vi "uDaq.vi"() -> (0 "error out":errorcluster)   [LabVIEW 2017]
uses:
  <vilib>/Platform/TimedLoop/XDataNode/timing_clust.ctl
  <vilib>/Platform/TimedLoop/XDataNode/nitl_modes.ctl
  <vilib>/Platform/TimedLoop/XDataNode/wakeup.ctl
  Globals/measurementGlobal.vi
  <vilib>/platform/TimedLoop/XDataNode/XDataNode.xnode
  <vilib>/Platform/TimedLoop/XDataNode/XDNodeRunTimeDep.lvlib
panel:
  out "Analogue Data (volts?)":dbl[][](array[numeric])
  out "Block Index":i32
  out "Case":string[](array[string])
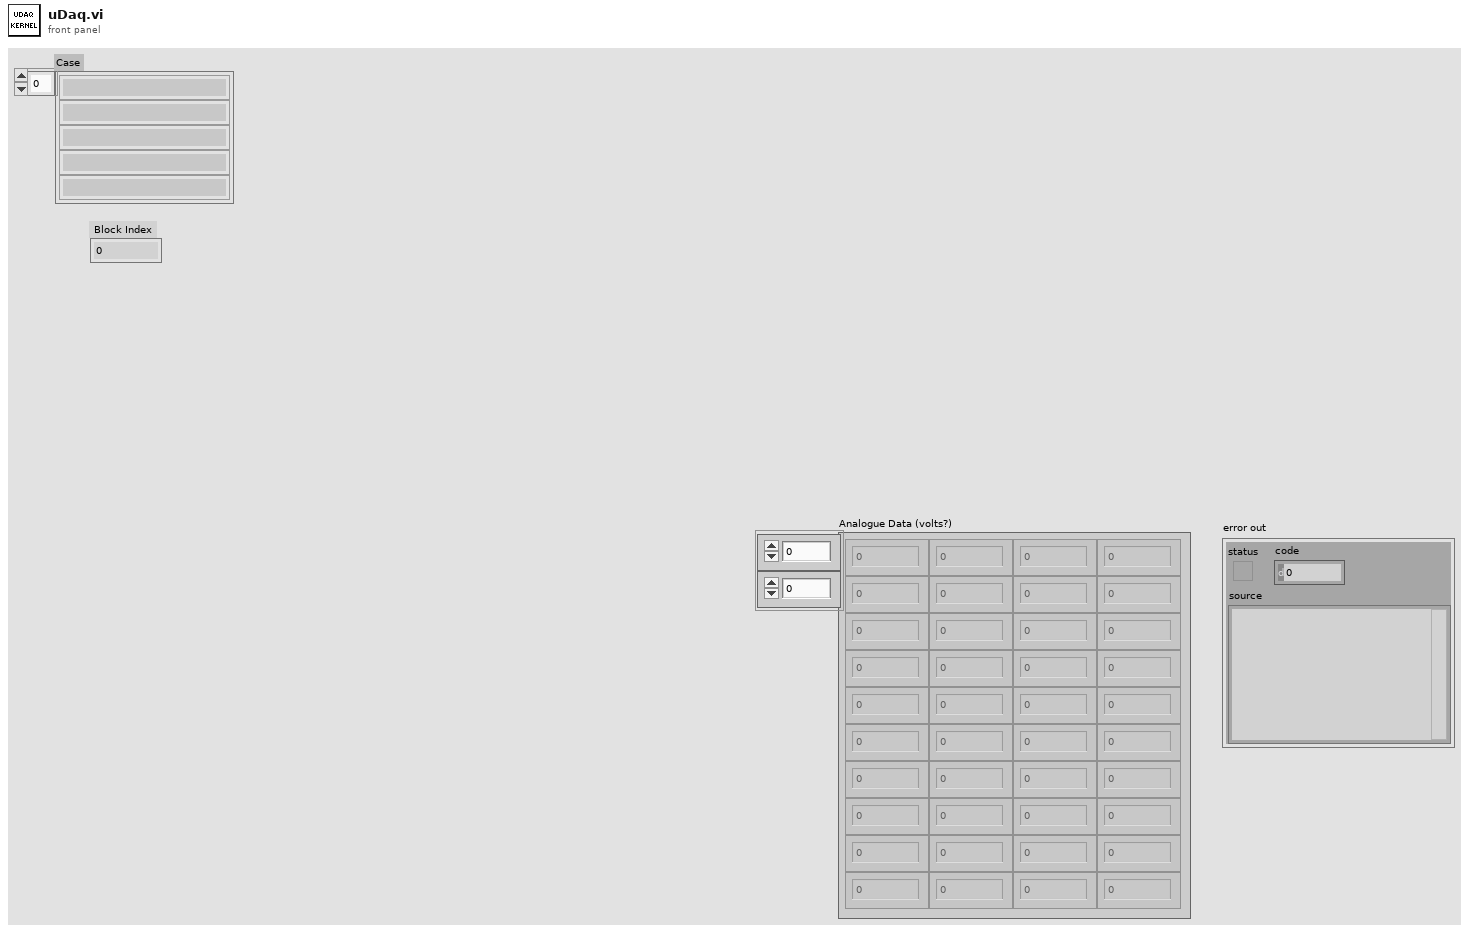
[diagram p1: front panel]
types:
  T1 = typedef "XDNodeRunTimeDep.lvlib/timing_clust.ctl" = cluster{"Expected End [f-1]":u64, "Actual End [f-1]":u64, "Finished Late? [f-1]":bool, "Expected End [i-1]":u64, "Actual End [i-1]":u64, "Finished Late? [i-1]":bool, "Expected Start [i]":u64, "Actual Start [i]":u64, "Expected Start [f]":u64, "Actual Start [f]":u64, "Source Name":string, "Structure Name":string, "Period":i64, "Deadline":i64, "Offset":i64, "Start":i64, "Priority":i32, "Timeout":i32, "Mode":T2, "Wakeup Reason":T3, "Error":errorcluster, "Source Type":string, "Secondary Source Type":string, "Global End Time":u64, "Global Start Time":u64, "Frame Duration":u64, "Iteration Duration":u64, "Assigned CPU":i32, "I/O Scan Engine Mode":u32}
  T2 = typedef "XDNodeRunTimeDep.lvlib/nitl_modes.ctl" = enum32{"No Change", "Process missed periods, maintain original phase", "Discard missed periods, maintain original phase", "Process missed periods, ignore original phase", "Discard missed periods, ignore original phase"}
  T3 = typedef "XDNodeRunTimeDep.lvlib/wakeup.ctl" = enum32{"Normal", "Aborted", "Asynchronous wakeup", "Timing source error", "Timed loop error", "Timeout"}
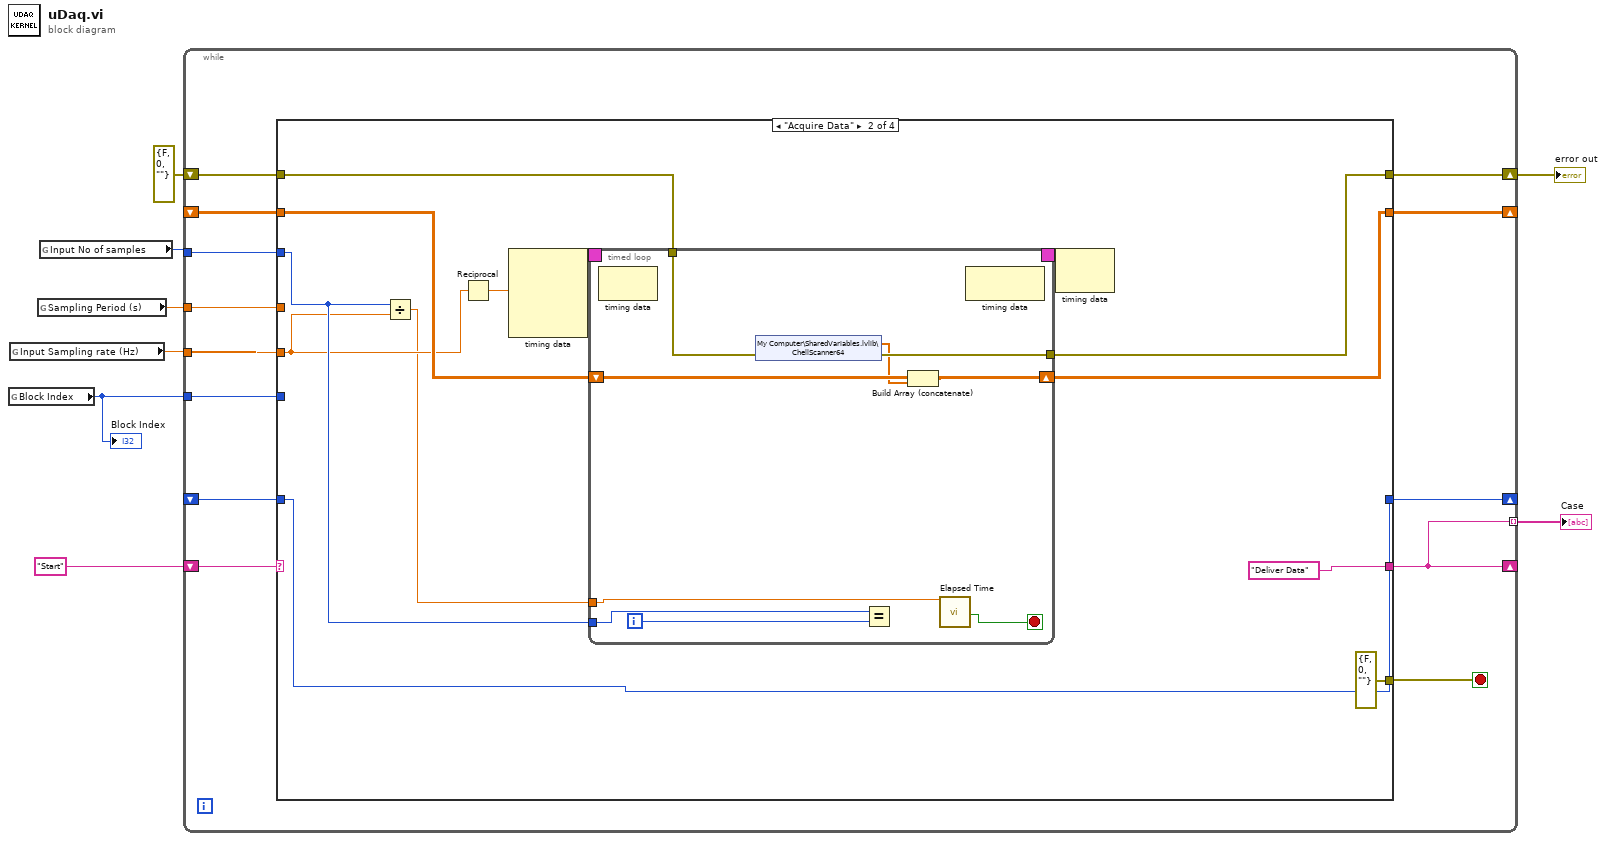
[diagram p0: block diagram]
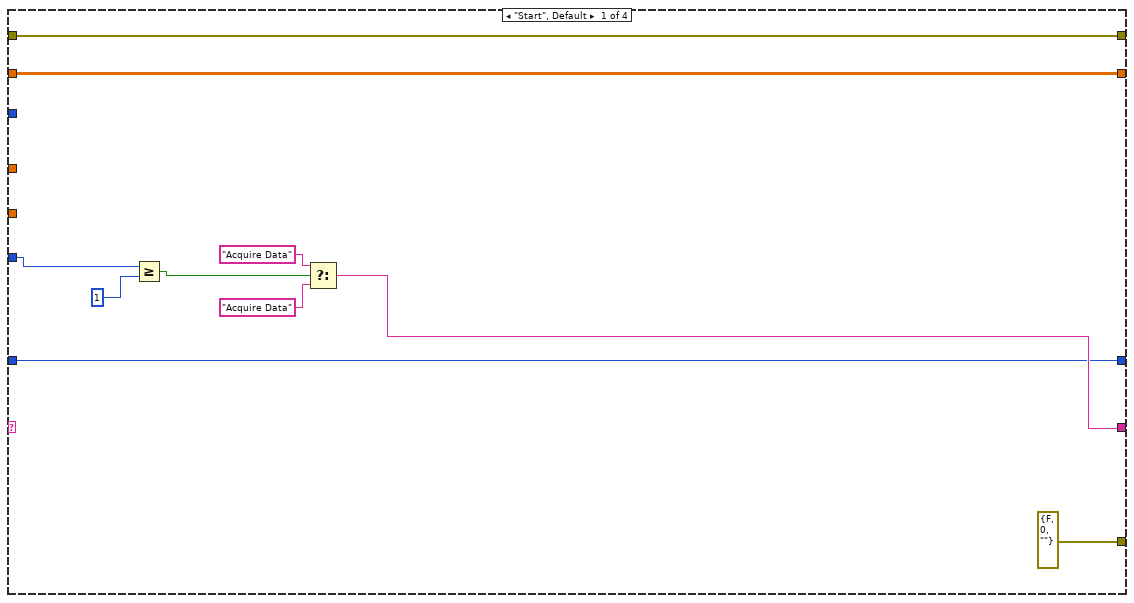
[diagram p2: hidden frame]
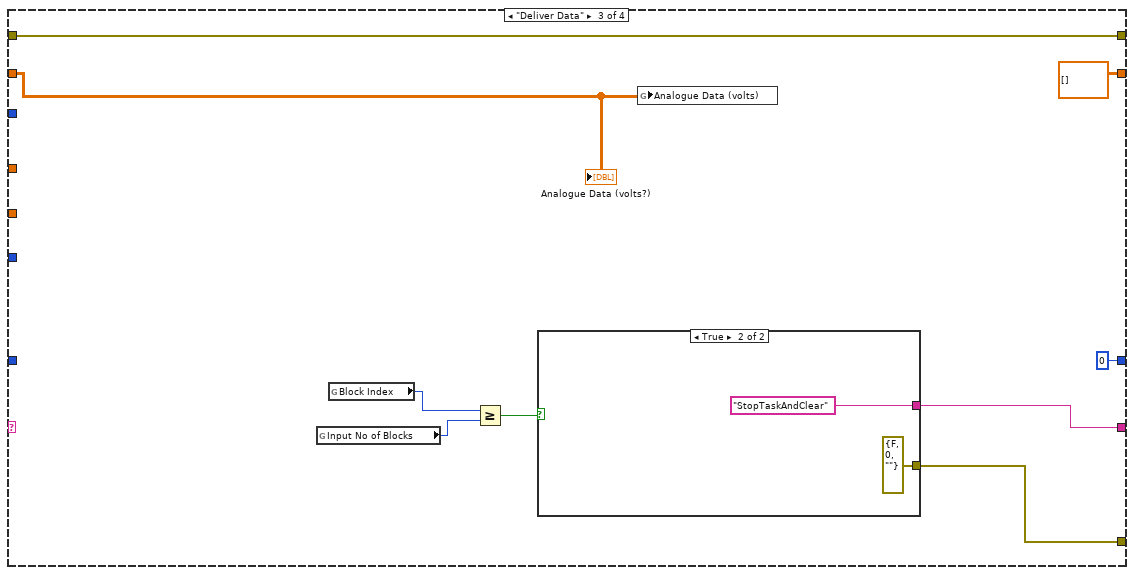
[diagram p3: hidden frame]
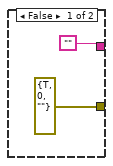
[diagram p4: hidden frame]
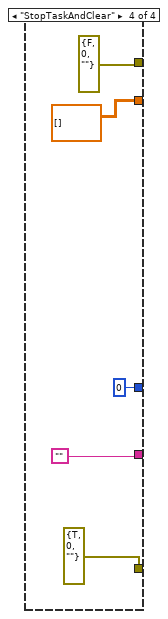
[diagram p5: hidden frame]
diagram:
  n1 = global read "measurementGlobal.vi" "Block Index"() -> (w2:i32)
  "Block Index" <- w2
  n2 = global read "measurementGlobal.vi" "Input Sampling rate (Hz)"() -> (w7:dbl)
  n3 = global read "measurementGlobal.vi" "Sampling Period (s)"() -> (w3:dbl)
  n4 = global read "measurementGlobal.vi" "Input No of samples"() -> (w8:i32)
  n5 = while {
    tunnel: w8 -> [w21]
    tunnel: w7 -> [w20]
    shift-right: [w19] -> w6
    shift-left: errorcluster {"status"=FALSE, "code"=0, "source"=""} ("error out") -> [w18]
    shift-right: [w13] -> _
    shift-left: _ -> [w16]
    shift-right: [w14] -> _
    shift-left: "Start" -> [w15]
    tunnel: [w14] -> w4 mode=indexing
    tunnel: w3 -> [w12]
    shift-right: [w10] -> _
    shift-left: _ -> [w11]
    tunnel: w2 -> [w9]
    stop <- w17 stop-if-true
    n6 = case shown="\"Acquire Data\"" w15 {
      tunnel: w21 -> [_ w35 _ _]
      tunnel: w20 -> [_ w34 _ _]
      tunnel: [w26 w40 w68 errorcluster {"status"=FALSE, "code"=0, "source"=""} ("error out")] -> w19
      tunnel: w18 -> [w26 w41 w68 _]
      tunnel: [errorcluster {"status"=FALSE, "code"=0, "source"=""} ("error out") errorcluster {"status"=FALSE, "code"=0, "source"=""} ("error out") w61 errorcluster {"status"=TRUE, "code"=0, "source"=""} ("error out")] -> w17
      tunnel: [w31 w38 dbl[][] [] ("data") dbl[][] [] ("data")] -> w13
      tunnel: w16 -> [w31 w37 w60 _]
      tunnel: [w27 "Deliver Data" w65 ""] -> w14
      tunnel: w12 -> [_ _ _ _]
      tunnel: w11 -> [w24 w44 _ _]
      tunnel: [w24 w44 0 0] -> w10
      tunnel: w9 -> [w23 _ _ _]
      frame "Start", Default {
        n7 = Greater Or Equal?(x=w23, y=1) -> (x >= y?=w29:bool)
        n8 = Select(t="Acquire Data" ("f"), s=w29, f="Acquire Data") -> (s? t:f=w27:string)
      }
      frame "Acquire Data" {
        n9 = Divide(x=w35, y=w34) -> (x/y=w32:dbl)
        n10 = Reciprocal(x=w34) -> (1/x=w33:dbl)
        n11 = node-c288(w33) -> (w43:T1)  [unwired: 3 in]
        n12 = timed-loop {
          timing: w43 -> [_]
          timing-out: [_] -> w42
          tunnel: w41 -> [w53]
          tunnel: [w52] -> w40
          shift-right: [w51] -> w38
          shift-left: w37 -> [w50]
          tunnel: w35 -> [w47]
          tunnel: w32 -> [w49]
          i -> [w48]
          stop <- w46 stop-if-true
          n13 = node-c288() -> ()  [unwired: 1 in, 1 out]
          n14 = shared-variable "My Computer\\SharedVariables.lvlib\\ChellScanner64"(error in=w53) -> (w45:dbl[], error out=w52:errorcluster)
          n15 = Equal?(x=w47, y=w48) -> ()  [unwired: 1 out]
          n16 = Build Array (concatenate)(w50, w45) -> (w51:dbl[][])
          n17 = call "Elapsed Time"("Time Target (s)"=w49) -> ("Time has Elapsed"=w46:bool)  [unwired: 11 in, 7 out]
          n18 = node-c288() -> ()  [unwired: 1 in, 1 out]
        }
        n19 = node-c288(w42) -> ()  [unwired: 1 out]
      }
      frame "Deliver Data" {
        n20 = global read "measurementGlobal.vi" "Input No of Blocks"() -> (w67:i32)
        n21 = global read "measurementGlobal.vi" "Block Index"() -> (w62:i32)
        n22 = Greater Or Equal?(x=w62, y=w67) -> (x >= y?=w66:bool)
        n23 = case shown="True" w66 {
          tunnel: ["" "StopTaskAndClear"] -> w65
          tunnel: [errorcluster {"status"=TRUE, "code"=0, "source"=""} ("error out") errorcluster {"status"=FALSE, "code"=0, "source"=""} ("error out")] -> w61
          frame False {
          }
          frame True {
          }
        }
        n24 = global write "measurementGlobal.vi" "Analogue Data (volts)"(w60) -> ()
        "Analogue Data (volts?)" <- w60
      }
      frame "StopTaskAndClear" {
      }
    }
  }
  "error out" <- w6
  "Case" <- w4
